vi "test-setValue2.vi"() -> ()   [LabVIEW 2019, in "lv-apt-json-file-test.lvlib"]
uses:
  lv-apt-json-file-test.lvlib
  Def-AttrMap.ctl
  lv-apt-json-file.lvlib
panel:
  out "OrignKey":string
  out "Variant":variant
  out "AttrMap out":T1
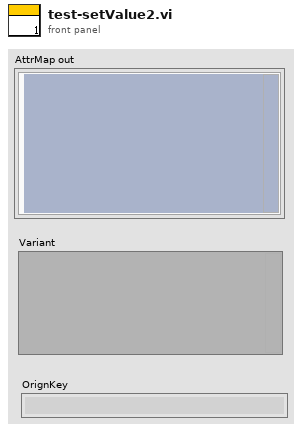
[diagram p1: front panel]
types:
  T1 = typedef "lv-apt-json-file.lvlib/Def-AttrMap.ctl" = cluster{"Map":variant}
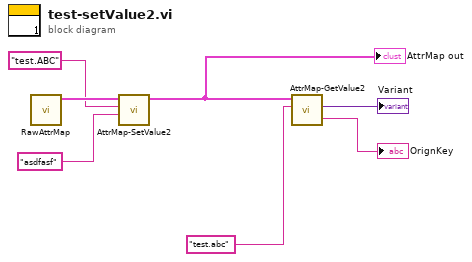
[diagram p0: block diagram]
diagram:
  n1 = call "RawAttrMap.vi"() -> ("AttrMap"=w7:T1)  [unwired: 11 in]
  n2 = call "AttrMap-SetValue2.vi"("Value"="asdfasf", "Key"="test.ABC", "AttrMap in"=w7) -> ("AttrMap out"=w5:T1)  [unwired: 7 in, 1 out]
  "AttrMap out" <- w5
  n3 = call "AttrMap-GetValue2.vi"("Key"="test.abc", "AttrMap in"=w5) -> ("Variant"=→"Variant":variant, "OrignKey"=→"OrignKey":string)  [unwired: 6 in, 2 out]
